vi "Data Replay Page.vi"(8 "error in (no error)":errorcluster, 11 "Node Ptr":T3 format="%.0x") -> (0 "error out":errorcluster)   [LabVIEW 2011, in "Engine Sim System Explorer.lvlib"]
uses:
  Engine Sim System Explorer.lvlib
  <vilib>/NI Veristand/Custom Device API/Custom Device Item Ref.ctl
  TypeDefs/FPGA Mem Size.ctl
  TypeDefs/AngleReference.ctl
  <vilib>/NI Veristand/Custom Device API/Custom Device Channel.ctl
  <vilib>/NI Veristand/Custom Device API/Custom Device Channel Type.ctl
  Shared/Engine Simulation Global.vi
  <vilib>/NI Veristand/Custom Device API/Get Item Property (Boolean).vi
  <vilib>/NI Veristand/Custom Device API/Get Item Property (Double).vi
  <vilib>/NI Veristand/Custom Device API/Get Item Property (U16).vi
  <vilib>/NI Veristand/Custom Device API/Get Item Property (I32).vi
  <vilib>/NI Veristand/Custom Device API/Set Item Property (U16).vi
  <vilib>/NI Veristand/Custom Device API/Set Item Property (Boolean).vi
  <vilib>/NI Veristand/Custom Device Tools/Custom Device Utility Library/NI VeriStand - Search for Item by Name.vi
  <vilib>/NI Veristand/Custom Device API/Set Item Property (Double).vi
  <vilib>/NI Veristand/Custom Device API/Custom Device API.lvlib
  Engine Simulation Shared.lvlib
  <vilib>/NI Veristand/Custom Device Tools/Custom Device Utility Library/Custom Device Utility Library.lvlib
panel:
  in  "Tab Control":enum32{"Data", "Voltage", "Advanced"}(tab)
  in  "Refresh Graph":bool
  in  "CycleAngle?":T1 caption="FPGA simulation angle reference"
  out "Data Graph":waveform(dbl)(graph)
  in  "FPGA memory size":T2
  in  "Load":bool
  in  "VOverride":bool
  in  "ReverseNegate":bool
  out "Voltage XY":cluster{dbl, dbl}[](graph)
  in  "Voltage at maximum speed":dbl=1.0 min=0.0 max=10.0
  in  "Voltage at cutoff speed":dbl=1.0 min=0.0 max=10.0
  in  "Cutoff speed (RPM)":dbl=1.0 min=0.0
  in  "Maximum speed (RPM)":dbl=1.0 min=1.0
  in  "DAC Bits":u16=1 min=1 max=16
  out "FPGA Memory #":i32
  in  "SHDocVw.IWebBrowser2":refnum<k7>(container)
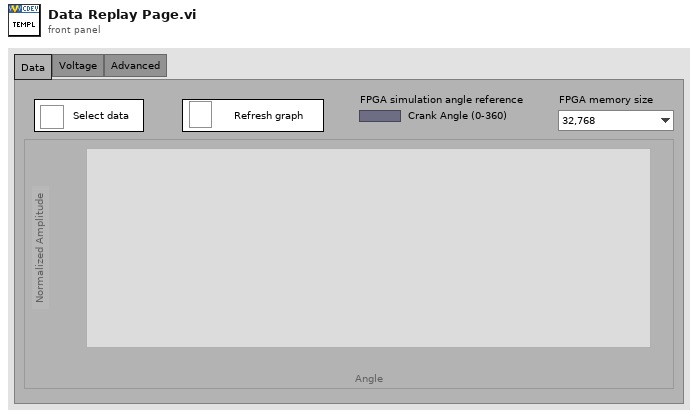
[diagram p1: front panel]
types:
  T1 = typedef "Engine Sim System Explorer.lvlib/AngleReference.ctl" = bool
  T2 = typedef "Engine Sim System Explorer.lvlib/FPGA Mem Size.ctl" = enum16{"32,768", "16,384", "8,192", "4,096", "2,048", "1024", "512", "256", "128"}
  T3 = typedef "Custom Device API.lvlib/Custom Device Item Ref.ctl" = u64
  T4 = enum8{"Enabled", "Disabled", "Disabled and Grayed Out"}
  T5 = typedef "Custom Device API.lvlib/Custom Device Channel.ctl" = cluster{"Type":T6, "Units":string, "Default Value":dbl, "Faultable":bool, "Scalable":bool}
  T6 = typedef "Custom Device API.lvlib/Custom Device Channel Type.ctl" = enum16{"Input", "Output"}
  T7 = typedef "Custom Device API.lvlib/Custom Device Commands.ctl" = enum16{"Default", "Item renamed", "Shutdown", "Dynamic button pressed"}
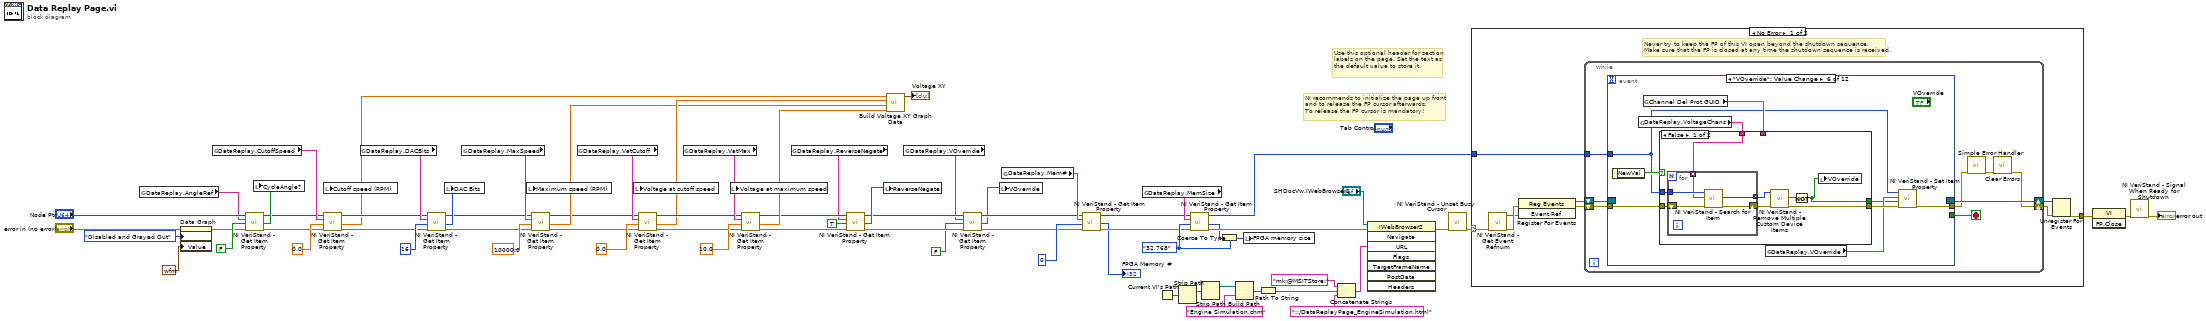
[diagram p0: block diagram]
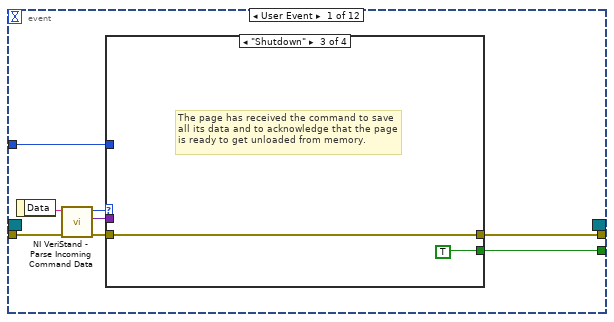
[diagram p2: hidden frame]
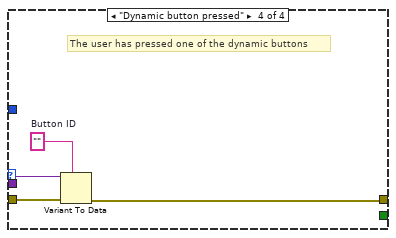
[diagram p5: hidden frame]
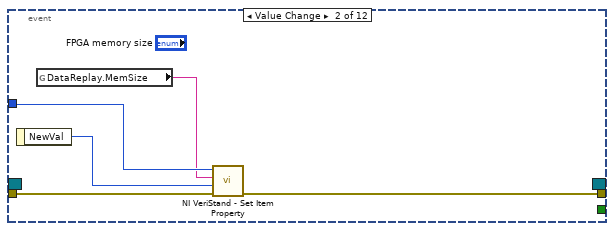
[diagram p6: hidden frame]
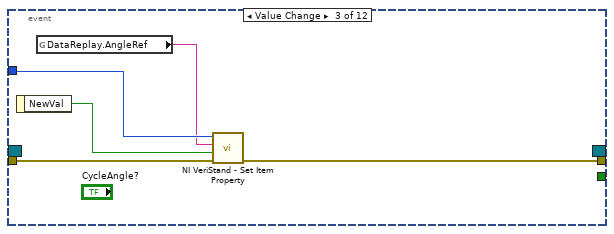
[diagram p7: hidden frame]
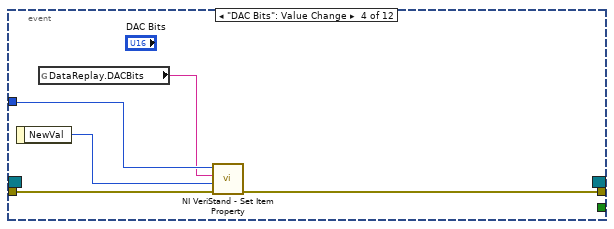
[diagram p8: hidden frame]
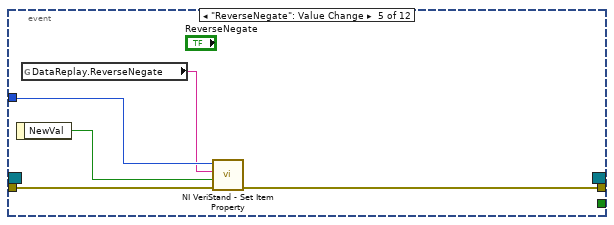
[diagram p9: hidden frame]
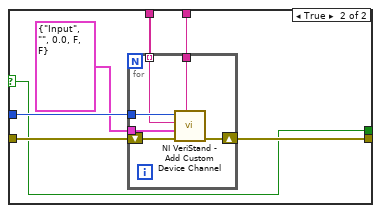
[diagram p10: hidden frame]
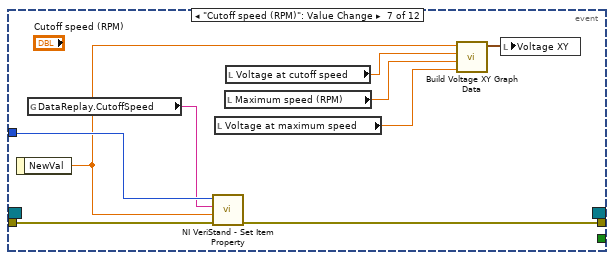
[diagram p11: hidden frame]
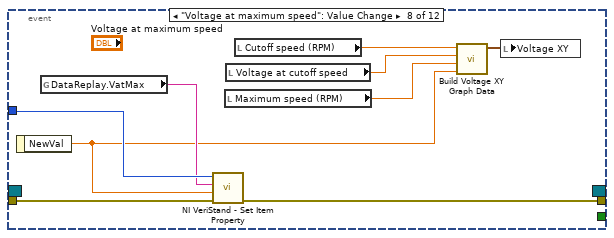
[diagram p12: hidden frame]
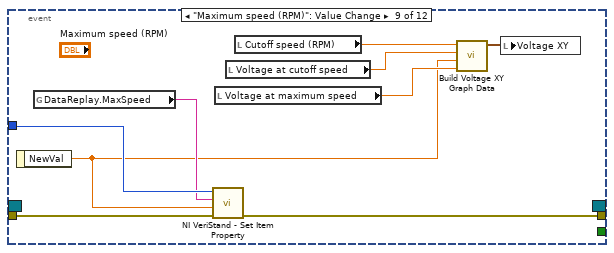
[diagram p13: hidden frame]
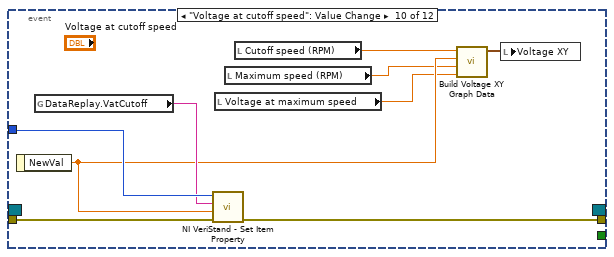
[diagram p14: hidden frame]
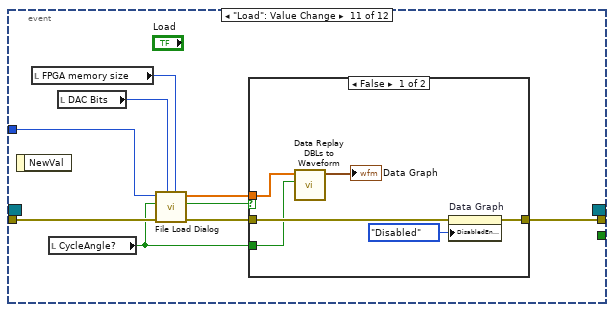
[diagram p15: hidden frame]
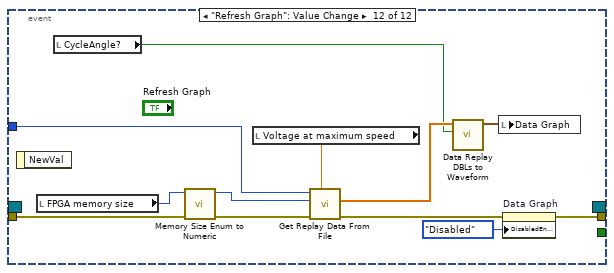
[diagram p17: hidden frame]
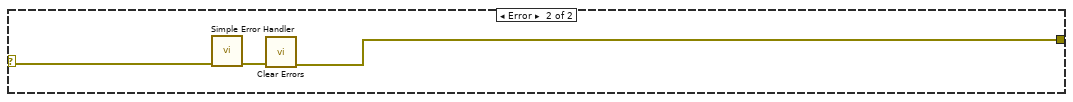
[diagram p18: hidden frame]
diagram:
  w53 = FPGA_Mem_Size."32,768" ("FPGA Memory Size")
  # "Use this optional header for section labels on the page. Set the text as the default value to store it."
  # "NI recommends to initialize the page up front\nand to release the FP cursor afterwards.\nTo release the FP cursor is mandatory!"
  n1 = global read "Engine Simulation Global.vi" "DataReplay.AngleRef"() -> (w44:string)
  n2 = property on="Data Graph" class="WFGraph (strict)"(error in="error in (no error)", "DisabledEnum"=T4."Disabled and Grayed Out" ("Disabled"), "Value"=waveform(dbl) {"t0"=timestamp(0 s since 1904-01-01), "dt"=1.0, "Y"=[]} ("Data Graph")) -> (error out=w14:errorcluster)  [unwired: 1 in, 1 out]
  n3 = global read "Engine Simulation Global.vi" "DataReplay.CutoffSpeed"() -> (w40:string)
  n4 = call-poly <vilib>:"NI VeriStand - Get Item Property.vi"("error in (no error)"=w14, "Default Value"=FALSE, "Property Name"=w44, "Item Ref in"="Node Ptr") -> ("error out"=w38:errorcluster, "Value"=w42:bool, "Item Ref out"=w39:T3)  [unwired: 4 in, 1 out]
  n5 = local write "CycleAngle?"(w42) -> ()
  n6 = call-poly <vilib>:"NI VeriStand - Get Item Property.vi"("error in (no error)"=w38, "Default Value"=0.0, "Property Name"=w40, "Item Ref in"=w39) -> ("error out"=w34:errorcluster, "Value"=w21:dbl, "Item Ref out"=w33:T3)  [unwired: 4 in, 1 out]
  n7 = local write "Cutoff speed (RPM)"(w21) -> ()
  n8 = global read "Engine Simulation Global.vi" "DataReplay.DACBits"() -> (w37:string)
  n9 = call-poly <vilib>:"NI VeriStand - Get Item Property.vi"("error in (no error)"=w34, "Default Value"=u16 16, "Property Name"=w37, "Item Ref in"=w33) -> ("error out"=w29:errorcluster, "Value"=w35:u16, "Item Ref out"=w30:T3)  [unwired: 4 in, 1 out]
  n10 = local write "DAC Bits"(w35) -> ()
  n11 = global read "Engine Simulation Global.vi" "DataReplay.MaxSpeed"() -> (w31:string)
  n12 = call-poly <vilib>:"NI VeriStand - Get Item Property.vi"("error in (no error)"=w29, "Default Value"=10000.0, "Property Name"=w31, "Item Ref in"=w30) -> ("error out"=w15:errorcluster, "Value"=w18:dbl, "Item Ref out"=w16:T3)  [unwired: 4 in, 1 out]
  n13 = local write "Maximum speed (RPM)"(w18) -> ()
  n14 = global read "Engine Simulation Global.vi" "DataReplay.VatCutoff"() -> (w27:string)
  n15 = call-poly <vilib>:"NI VeriStand - Get Item Property.vi"("error in (no error)"=w15, "Default Value"=0.0, "Property Name"=w27, "Item Ref in"=w16) -> ("error out"=w23:errorcluster, "Value"=w19:dbl, "Item Ref out"=w24:T3)  [unwired: 4 in, 1 out]
  n16 = local write "Voltage at cutoff speed"(w19) -> ()
  n17 = global read "Engine Simulation Global.vi" "DataReplay.VatMax"() -> (w26:string)
  n18 = call-poly <vilib>:"NI VeriStand - Get Item Property.vi"("error in (no error)"=w23, "Default Value"=10.0, "Property Name"=w26, "Item Ref in"=w24) -> ("error out"=w22:errorcluster, "Value"=w17:dbl, "Item Ref out"=w10:T3)  [unwired: 4 in, 1 out]
  n19 = local write "Voltage at maximum speed"(w17) -> ()
  n20 = global read "Engine Simulation Global.vi" "DataReplay.ReverseNegate"() -> (w9:string)
  n21 = call-poly <vilib>:"NI VeriStand - Get Item Property.vi"("error in (no error)"=w22, "Default Value"=TRUE, "Property Name"=w9, "Item Ref in"=w10) -> ("error out"=w11:errorcluster, "Value"=w8:bool, "Item Ref out"=w5:T3)  [unwired: 4 in, 1 out]
  n22 = local write "ReverseNegate"(w8) -> ()
  n23 = call "Build Voltage XY Graph Data.vi"("maximum voltage"=w17, "maximum speed"=w18, "cutoff voltage"=w19, "cutoff speed"=w21) -> ("XY data"=→"Voltage XY":cluster{dbl, dbl}[])  [unwired: 7 in]
  n24 = global read "Engine Simulation Global.vi" "DataReplay.VOverride"() -> (w3:string)
  n25 = call-poly <vilib>:"NI VeriStand - Get Item Property.vi"("error in (no error)"=w11, "Default Value"=FALSE, "Property Name"=w3, "Item Ref in"=w5) -> ("error out"=w6:errorcluster, "Value"=w2:bool, "Item Ref out"=w4:T3)  [unwired: 4 in, 1 out]
  n26 = local write "VOverride"(w2) -> ()
  n27 = global read "Engine Simulation Global.vi" "DataReplay.Mem#"() -> (w49:string)
  n28 = call-poly <vilib>:"NI VeriStand - Get Item Property.vi"("error in (no error)"=w6, "Default Value"=0, "Property Name"=w49, "Item Ref in"=w4) -> ("error out"=w50:errorcluster, "Value"=→"FPGA Memory #":i32, "Item Ref out"=w51:T3)  [unwired: 4 in, 1 out]
  n29 = global read "Engine Simulation Global.vi" "DataReplay.MemSize"() -> (w55:string)
  n30 = Current VI's Path() -> (path=w62:path)
  n31 = Strip Path(path=w62) -> (stripped path=w63:path)  [unwired: 1 out]
  n32 = call-poly <vilib>:"NI VeriStand - Get Item Property.vi"("error in (no error)"=w50, "Default Value"=w53, "Property Name"=w55, "Item Ref in"=w51) -> ("error out"=w57:errorcluster, "Value"=w54:u16, "Item Ref out"=w56:T3)  [unwired: 4 in, 1 out]
  n33 = Strip Path(path=w63) -> (stripped path=w68:path)  [unwired: 1 out]
  n34 = Coerce To Type(0:w54, 1:w53) -> (2:w52:T2)
  n35 = Build Path(base path=w68, name or relative path="Engine Simulation.chm") -> (appended path=w66:path)
  n36 = local write "FPGA memory size"(w52) -> ()
  n37 = Path To String(path=w66) -> (string=w65:string)
  n38 = Concatenate Strings("mk:@MSITStore:" ("string"), w65, "::/DataReplayPage_EngineSimulation.html" ("name or relative path")) -> (w60:string)
  n39 = invoke class="IWebBrowser2" method="Navigate"(reference="SHDocVw.IWebBrowser2", error in=w57, "URL"=w60) -> (error out=w59:errorcluster)  [unwired: 5 in, 7 out]
  n40 = call <vilib>:"NI VeriStand - Unset Busy Cursor.vi"("error in (no error)"=w59) -> ("error out"=w69:errorcluster)  [unwired: 10 out]
  n41 = case shown="No Error" w69 {
    selector: w69 -> [w73 w227]
    tunnel: [w78 w225] -> w72
    tunnel: w56 -> [w74 _]
    frame No Error {
      # "Never try to keep the FP of this VI open beyond the shutdown sequence.\nMake sure that the FP is closed at any time the shutdown sequence is received."
      n42 = call <vilib>:"NI VeriStand - Get Event Refnum.vi"("error in (no error)"=w73) -> ("error out"=w81:errorcluster, "Event Ref"=w77:refnum<user-event>)  [unwired: 9 out]
      n43 = register-events(error in=w81, w77) -> (reference out=w75:refnum<event-registration>, error out=w76:errorcluster)  [unwired: 1 in]
      n44 = while {
        tunnel: w74 -> [w85]
        shift-right: [w82] -> w79
        shift-left: w76 -> [w88]
        shift-right: [w89] -> w80
        shift-left: w75 -> [w87]
        stop <- w86 stop-if-true
        n45 = event shown="[5] \"VOverride\": Value Change" {
          selector: w87 -> [_ _ _ _ _ _ _ _ _ _ _ _]
          dyn-events: [_ _ _ _ _ _ _ _ _ _ _ _] -> w89
          timeout: _ -> [_ _ _ _ _ _ _ _ _ _ _ _]
          tunnel: w88 -> [w97 w110 w115 w120 w125 w131 w169 w178 w187 w196 w205 w216]
          tunnel: [w93 _ _ _ _ _ _ _ _ _ _ _] -> w86
          tunnel: [w92 w106 w111 w116 w121 w129 w166 w175 w184 w193 w204 w223] -> w84
          tunnel: w85 -> [w91 w109 w114 w119 w124 w128 w168 w177 w186 w195 w201 w221]
          event User Event {
            n46 = event-data() -> ("Data"=w96:string)  [unwired: 1 out]
            n47 = call <vilib>:"NI VeriStand - Parse Incoming Command Data.vi"("error in (no error)"=w97, "Incoming data"=w96) -> ("error out"=w95:errorcluster, "Outgoing data"=w90:variant, "Action"=w94:T7)  [unwired: 7 out]
            n48 = case shown="\"Shutdown\"" w94 {
              tunnel: w95 -> [w98 w99 w100 w105]
              tunnel: [_ _ TRUE _] -> w93
              tunnel: [w98 w99 w100 w102] -> w92
              tunnel: w91 -> [_ _ _ _]
              tunnel: w90 -> [_ _ _ w104]
              frame "Default", Default {
              }
              frame "Item renamed" {
              }
              frame "Shutdown" {
                # "The page has received the command to save all its data and to acknowledge that the page is ready to get unloaded from memory."
              }
              frame "Dynamic button pressed" {
                w103 = ""  # Button ID
                # "The user has pressed one of the dynamic buttons"
                n49 = Variant To Data(error in=w105, type=w103, Variant=w104) -> (error out=w102:errorcluster)  [unwired: 1 out]
              }
            }
          }
          event Value Change {
            n50 = event-data() -> ("NewVal"=w108:T2)  [unwired: 1 out]
            n51 = global read "Engine Simulation Global.vi" "DataReplay.MemSize"() -> (w107:string)
            n52 = call-poly <vilib>:"NI VeriStand - Set Item Property.vi"("error in (no error)"=w110, "Value"=w108, "Property Name"=w107, "Item Ref in"=w109) -> ("error out"=w106:errorcluster)  [unwired: 5 in, 2 out]
          }
          event Value Change {
            n53 = event-data() -> ("NewVal"=w113:T1)  [unwired: 1 out]
            n54 = global read "Engine Simulation Global.vi" "DataReplay.AngleRef"() -> (w112:string)
            n55 = call-poly <vilib>:"NI VeriStand - Set Item Property.vi"("error in (no error)"=w115, "Value"=w113, "Property Name"=w112, "Item Ref in"=w114) -> ("error out"=w111:errorcluster)  [unwired: 5 in, 2 out]
          }
          event "DAC Bits": Value Change {
            n56 = event-data() -> ("NewVal"=w118:u16)  [unwired: 1 out]
            n57 = global read "Engine Simulation Global.vi" "DataReplay.DACBits"() -> (w117:string)
            n58 = call-poly <vilib>:"NI VeriStand - Set Item Property.vi"("error in (no error)"=w120, "Value"=w118, "Property Name"=w117, "Item Ref in"=w119) -> ("error out"=w116:errorcluster)  [unwired: 5 in, 2 out]
          }
          event "ReverseNegate": Value Change {
            n59 = event-data() -> ("NewVal"=w123:bool)  [unwired: 1 out]
            n60 = global read "Engine Simulation Global.vi" "DataReplay.ReverseNegate"() -> (w122:string)
            n61 = call-poly <vilib>:"NI VeriStand - Set Item Property.vi"("error in (no error)"=w125, "Value"=w123, "Property Name"=w122, "Item Ref in"=w124) -> ("error out"=w121:errorcluster)  [unwired: 5 in, 2 out]
          }
          event "VOverride": Value Change {
            n62 = event-data() -> ("NewVal"=w134:bool)  [unwired: 1 out]
            n63 = global read "Engine Simulation Global.vi" "DataReplay.VoltageChans"() -> (w133:string[])
            n64 = global read "Engine Simulation Global.vi" "Channel Del Prot GUID"() -> (w132:string)
            n65 = case shown="False" w134 {
              selector: w134 -> [_ w148]
              tunnel: w131 -> [w142 w154]
              tunnel: w128 -> [w141 w153]
              tunnel: w133 -> [w140 w152]
              tunnel: w132 -> [_ w151]
              tunnel: [w136 w149] -> w130
              tunnel: [w135 w148] -> w126
              frame False {
                n66 = for {
                  tunnel: w141 -> [w146]
                  tunnel: w140 -> [w145] mode=indexing
                  shift-right: [w144] -> w139
                  shift-left: w142 -> [w147]
                  tunnel: [w143] -> w138 mode=indexing
                  n67 = call-poly <vilib>:"NI VeriStand - Search for Item.vi"("error in"=w147, "Item Name"=w145, "Section Ref in"=w146) -> ("error out"=w144:errorcluster, "Item Ref"=w143:T3)  [unwired: 5 in, 2 out]
                }
                n68 = call <vilib>:"NI VeriStand - Remove Multiple Custom Device Items.vi"("error in (no error)"=w139, "Item Refs in"=w138) -> ("error out"=w136:errorcluster, "Deleted?"=w137:bool)  [unwired: 8 in]
                n69 = Not(x=w137) -> (.not. x?=w135:bool)
                n70 = local write "VOverride"(w135) -> ()
              }
              frame True {
                n71 = for {
                  shift-right: [w159] -> w149
                  shift-left: w154 -> [w160]
                  tunnel: w153 -> [w158]
                  tunnel: w152 -> [w157] mode=indexing
                  tunnel: w151 -> [w156]
                  tunnel: T5 {"Type"=enum."Input", "Units"="", "Default Value"=0.0, "Faultable"=FALSE, "Scalable"=FALSE} ("Channel") -> [w155]
                  n72 = call <vilib>:"NI VeriStand - Add Custom Device Channel.vi"("GUID (Default Channel)"=w156, "error in (no error)"=w160, "Channel"=w155, "Channel Name"=w157, "Parent Ref in"=w158) -> ("error out"=w159:errorcluster)  [unwired: 3 in, 3 out]
                }
              }
            }
            n73 = global read "Engine Simulation Global.vi" "DataReplay.VOverride"() -> (w127:string)
            n74 = call-poly <vilib>:"NI VeriStand - Set Item Property.vi"("error in (no error)"=w130, "Value"=w126, "Property Name"=w127, "Item Ref in"=w128) -> ("error out"=w129:errorcluster)  [unwired: 5 in, 2 out]
          }
          event "Cutoff speed (RPM)": Value Change {
            n75 = event-data() -> ("NewVal"=w161:dbl)  [unwired: 1 out]
            n76 = global read "Engine Simulation Global.vi" "DataReplay.CutoffSpeed"() -> (w167:string)
            n77 = call-poly <vilib>:"NI VeriStand - Set Item Property.vi"("error in (no error)"=w169, "Value"=w161, "Property Name"=w167, "Item Ref in"=w168) -> ("error out"=w166:errorcluster)  [unwired: 5 in, 2 out]
            n78 = local read "Voltage at maximum speed"() -> (w164:dbl)
            n79 = local read "Maximum speed (RPM)"() -> (w163:dbl)
            n80 = local read "Voltage at cutoff speed"() -> (w162:dbl)
            n81 = call "Build Voltage XY Graph Data.vi"("maximum voltage"=w164, "maximum speed"=w163, "cutoff voltage"=w162, "cutoff speed"=w161) -> ("XY data"=w165:cluster{dbl, dbl}[])  [unwired: 7 in]
            n82 = local write "Voltage XY"(w165) -> ()
          }
          event "Voltage at maximum speed": Value Change {
            n83 = event-data() -> ("NewVal"=w170:dbl)  [unwired: 1 out]
            n84 = global read "Engine Simulation Global.vi" "DataReplay.VatMax"() -> (w176:string)
            n85 = call-poly <vilib>:"NI VeriStand - Set Item Property.vi"("error in (no error)"=w178, "Value"=w170, "Property Name"=w176, "Item Ref in"=w177) -> ("error out"=w175:errorcluster)  [unwired: 5 in, 2 out]
            n86 = local read "Maximum speed (RPM)"() -> (w171:dbl)
            n87 = local read "Voltage at cutoff speed"() -> (w172:dbl)
            n88 = local read "Cutoff speed (RPM)"() -> (w173:dbl)
            n89 = call "Build Voltage XY Graph Data.vi"("maximum voltage"=w170, "maximum speed"=w171, "cutoff voltage"=w172, "cutoff speed"=w173) -> ("XY data"=w174:cluster{dbl, dbl}[])  [unwired: 7 in]
            n90 = local write "Voltage XY"(w174) -> ()
          }
          event "Maximum speed (RPM)": Value Change {
            n91 = event-data() -> ("NewVal"=w179:dbl)  [unwired: 1 out]
            n92 = global read "Engine Simulation Global.vi" "DataReplay.MaxSpeed"() -> (w185:string)
            n93 = call-poly <vilib>:"NI VeriStand - Set Item Property.vi"("error in (no error)"=w187, "Value"=w179, "Property Name"=w185, "Item Ref in"=w186) -> ("error out"=w184:errorcluster)  [unwired: 5 in, 2 out]
            n94 = local read "Voltage at maximum speed"() -> (w181:dbl)
            n95 = local read "Voltage at cutoff speed"() -> (w180:dbl)
            n96 = local read "Cutoff speed (RPM)"() -> (w182:dbl)
            n97 = call "Build Voltage XY Graph Data.vi"("maximum voltage"=w181, "maximum speed"=w179, "cutoff voltage"=w180, "cutoff speed"=w182) -> ("XY data"=w183:cluster{dbl, dbl}[])  [unwired: 7 in]
            n98 = local write "Voltage XY"(w183) -> ()
          }
          event "Voltage at cutoff speed": Value Change {
            n99 = event-data() -> ("NewVal"=w190:dbl)  [unwired: 1 out]
            n100 = global read "Engine Simulation Global.vi" "DataReplay.VatCutoff"() -> (w194:string)
            n101 = call-poly <vilib>:"NI VeriStand - Set Item Property.vi"("error in (no error)"=w196, "Value"=w190, "Property Name"=w194, "Item Ref in"=w195) -> ("error out"=w193:errorcluster)  [unwired: 5 in, 2 out]
            n102 = local read "Voltage at maximum speed"() -> (w189:dbl)
            n103 = local read "Maximum speed (RPM)"() -> (w188:dbl)
            n104 = local read "Cutoff speed (RPM)"() -> (w191:dbl)
            n105 = call "Build Voltage XY Graph Data.vi"("maximum voltage"=w189, "maximum speed"=w188, "cutoff voltage"=w190, "cutoff speed"=w191) -> ("XY data"=w192:cluster{dbl, dbl}[])  [unwired: 7 in]
            n106 = local write "Voltage XY"(w192) -> ()
          }
          event "Load": Value Change {
            n107 = event-data() -> ()  [unwired: 2 out]
            n108 = local read "FPGA memory size"() -> (w199:T2)
            n109 = local read "CycleAngle?"() -> (w197:T1)
            n110 = local read "DAC Bits"() -> (w200:u16)
            n111 = call "File Load Dialog.vi"("FPGA memory size"=w199, "DAC Bits"=w200, "error in (no error)"=w205, "CycleAngle?"=w197, "Node Ptr"=w201) -> ("error out"=w203:errorcluster, "Cancelled"=w202:bool, "Data"=w198:dbl[])  [unwired: 4 in]
            n112 = case shown="False" w202 {
              tunnel: [w210 w212] -> w204
              tunnel: w203 -> [w211 w212]
              tunnel: w198 -> [w208 _]
              tunnel: w197 -> [w207 _]
              frame False {
                n113 = call "Data Replay DBLs to Waveform.vi"("CycleAngle?"=w207, "Data"=w208) -> ("waveform"=→"Data Graph":waveform(dbl))  [unwired: 9 in]
                n114 = property on="Data Graph" class="WFGraph (strict)"(error in=w211, "DisabledEnum"=T4."Disabled" ("Disabled")) -> (error out=w210:errorcluster)  [unwired: 1 in, 1 out]
              }
              frame True {
              }
            }
          }
          event "Refresh Graph": Value Change {
            n115 = event-data() -> ()  [unwired: 2 out]
            n116 = local read "FPGA memory size"() -> (w215:T2)
            n117 = local read "CycleAngle?"() -> (w217:T1)
            n118 = call "Memory Size Enum to Numeric.vi"("error in (no error)"=w216, "FPGA Memory Size"=w215) -> ("error out"=w213:errorcluster, "Numeric"=w214:i32)  [unwired: 8 in]
            n119 = local read "Voltage at maximum speed"() -> (w220:dbl)
            n120 = call "Get Replay Data From File.vi"("V at Max RPM"=w220, "error in (no error)"=w213, "Memory Size (number)"=w214, "Item Ref in"=w221) -> ("error out"=w222:errorcluster, "DBL Data"=w218:dbl[])  [unwired: 5 in, 1 out]
            n121 = call "Data Replay DBLs to Waveform.vi"("CycleAngle?"=w217, "Data"=w218) -> ("waveform"=w219:waveform(dbl))  [unwired: 9 in]
            n122 = local write "Data Graph"(w219) -> ()
            n123 = property on="Data Graph" class="WFGraph (strict)"(error in=w222, "DisabledEnum"=T4."Disabled" ("Disabled")) -> (error out=w223:errorcluster)  [unwired: 1 in, 1 out]
          }
        }
        n124 = call <vilib>:"Simple Error Handler.vi"("error in (no error)"=w84) -> ("error out"=w83:errorcluster)  [unwired: 1 in, 7 out]
        n125 = call <vilib>:"Clear Errors.vi"("error in (no error)"=w83) -> ("error out"=w82:errorcluster)  [unwired: 6 out]
      }
      n126 = Unregister For Events(event registration refnum=w80, error in=w79) -> (error out=w78:errorcluster)
    }
    frame Error {
      n127 = call <vilib>:"Simple Error Handler.vi"("error in (no error)"=w227) -> ("error out"=w226:errorcluster)  [unwired: 1 in, 7 out]
      n128 = call <vilib>:"Clear Errors.vi"("error in (no error)"=w226) -> ("error out"=w225:errorcluster)  [unwired: 6 out]
    }
  }
  n129 = invoke class="VI" method="FP.Close"(error in=w72) -> (error out=w71:errorcluster)  [unwired: 2 in, 2 out]
  n130 = call <vilib>:"NI VeriStand - Signal When Ready for Shutdown.vi"("error in (no error)"=w71) -> ("error out"=→"error out":errorcluster)  [unwired: 10 out]
